vi "GetConfiguredSounds.vi"(11 "File":string="soundconfig.xml") -> (1 "Sound Cluster":T2={"Start"={"total number of samples/ch"=31680, "sound format"={"sample rate (S/s)"=11025.0, "number of channels"=1, "bits per sample"=16}, "data"=[{"t0"=timestamp(0 s since 1904-01-01), "dt"=9.070294784580499e-05, "Y"=array[31680 elements]}], "Volume"=100.0}, "Stop"={"total number of samples/ch"=27648, "sound format"={"sample rate (S/s)"=11025.0, "number of channels"=1, "bits per sample"=16}, "data"=[{"t0"=timestamp(0 s since 1904-01-01), "dt"=9.070294784580499e-05, "Y"=array[27648 elements]}], "Volume"=100.0}, "Uh-Oh"={"total number of samples/ch"=29952, "sound format"={"sample rate (S/s)"=11025.0, "number of channels"=1, "bits per sample"=16}, "data"=[{"t0"=timestamp(0 s since 1904-01-01), "dt"=9.070294784580499e-05, "Y"=array[29952 elements]}], "Volume"=88.46153846153847}, "PreMatch"={"total number of samples/ch"=225792, "sound format"={"sample rate (S/s)"=44100.0, "number of channels"=2, "bits per sample"=16}, "data"=[{"t0"=timestamp(0 s since 1904-01-01), "dt"=2.2675736961451248e-05, "Y"=array[225792 elements]}, {"t0"=timestamp(0 s since 1904-01-01), "dt"=2.2675736961451248e-05, "Y"=array[225792 elements]}], "Volume"=75.38461538461539}, "Hurry-Up"={"total number of samples/ch"=0, "sound format"={"sample rate (S/s)"=0.0, "number of channels"=0, "bits per sample"=0}, "data"=[], "Volume"=0.0}}, 3 "Settings Cluster":T1)   [LabVIEW 2013]
uses:
  Sound Info.ctl
  <vilib>/sound2/lvsound2.llb/Sound Data Format.ctl
  <vilib>/Utility/sysdir.llb/System Directory Type.ctl
  <vilib>/Utility/xml.llb/Read From XML File(string).vi
panel:
  in  "stop":bool
  out "output cluster":T1
  in  "Tab Control":enum32{"Page 1", "Page 2"}(tab)
  in  "Test Hurry Up Sound":bool
  in  "Load Hurry Up Sound":bool
  in  "Hurry Up Sound Volume":dbl(slide)=88.46153846153847 scale=0.0..100.0
  in  "Hurry Up Sound":path=path "C:/ProgramData/FLL/sounds/TimeToRun.wav"
  in  "Test Pre-Match Sound":bool
  in  "Load Pre-Match Sound":bool
  in  "Pre-Match Coundown Sound Volume":dbl(slide)=88.46153846153847 scale=0.0..100.0
  in  "Pre-Match Countdown Sound":path=path "Z:/Code/LabVIEW/FLL 2.1/sounds/FOGHORN.wav"
  in  "Test Uh-Oh Sound":bool
  in  "Load Uh-Oh Sound":bool
  in  "Uh-Oh Sound Volume":dbl(slide)=88.46153846153847 scale=0.0..100.0
  in  "Uh-Oh Sound Path":path=path "Z:/Code/LabVIEW/FLL 2.1/sounds/FOGHORN.wav"
  in  "Test Stop Sound":bool
  in  "Load Stop Sound":bool
  in  "Stop Sound Volume":dbl(slide)=100.0 scale=0.0..100.0
  in  "Stop Sound Path":path=path "Z:/Code/LabVIEW/FLL 2.1/sounds/BUZZER.wav"
  in  "Test Start Sound":bool
  in  "Load Start Sound":bool
  in  "Start Sound Volume":dbl(slide)=100.0 scale=0.0..100.0
  in  "Start Sound Path":path=path "Z:/Code/LabVIEW/FLL 2.1/sounds/CHARGE.wav"
  in  "Master Volume":dbl(slide)=100.0 min=1.0 scale=0.0..100.0
  in  "Secondary (s)":dbl
  in  "Primary (s)":dbl=150.0
  in  "Pre-Primary (s)":dbl
  # "5"
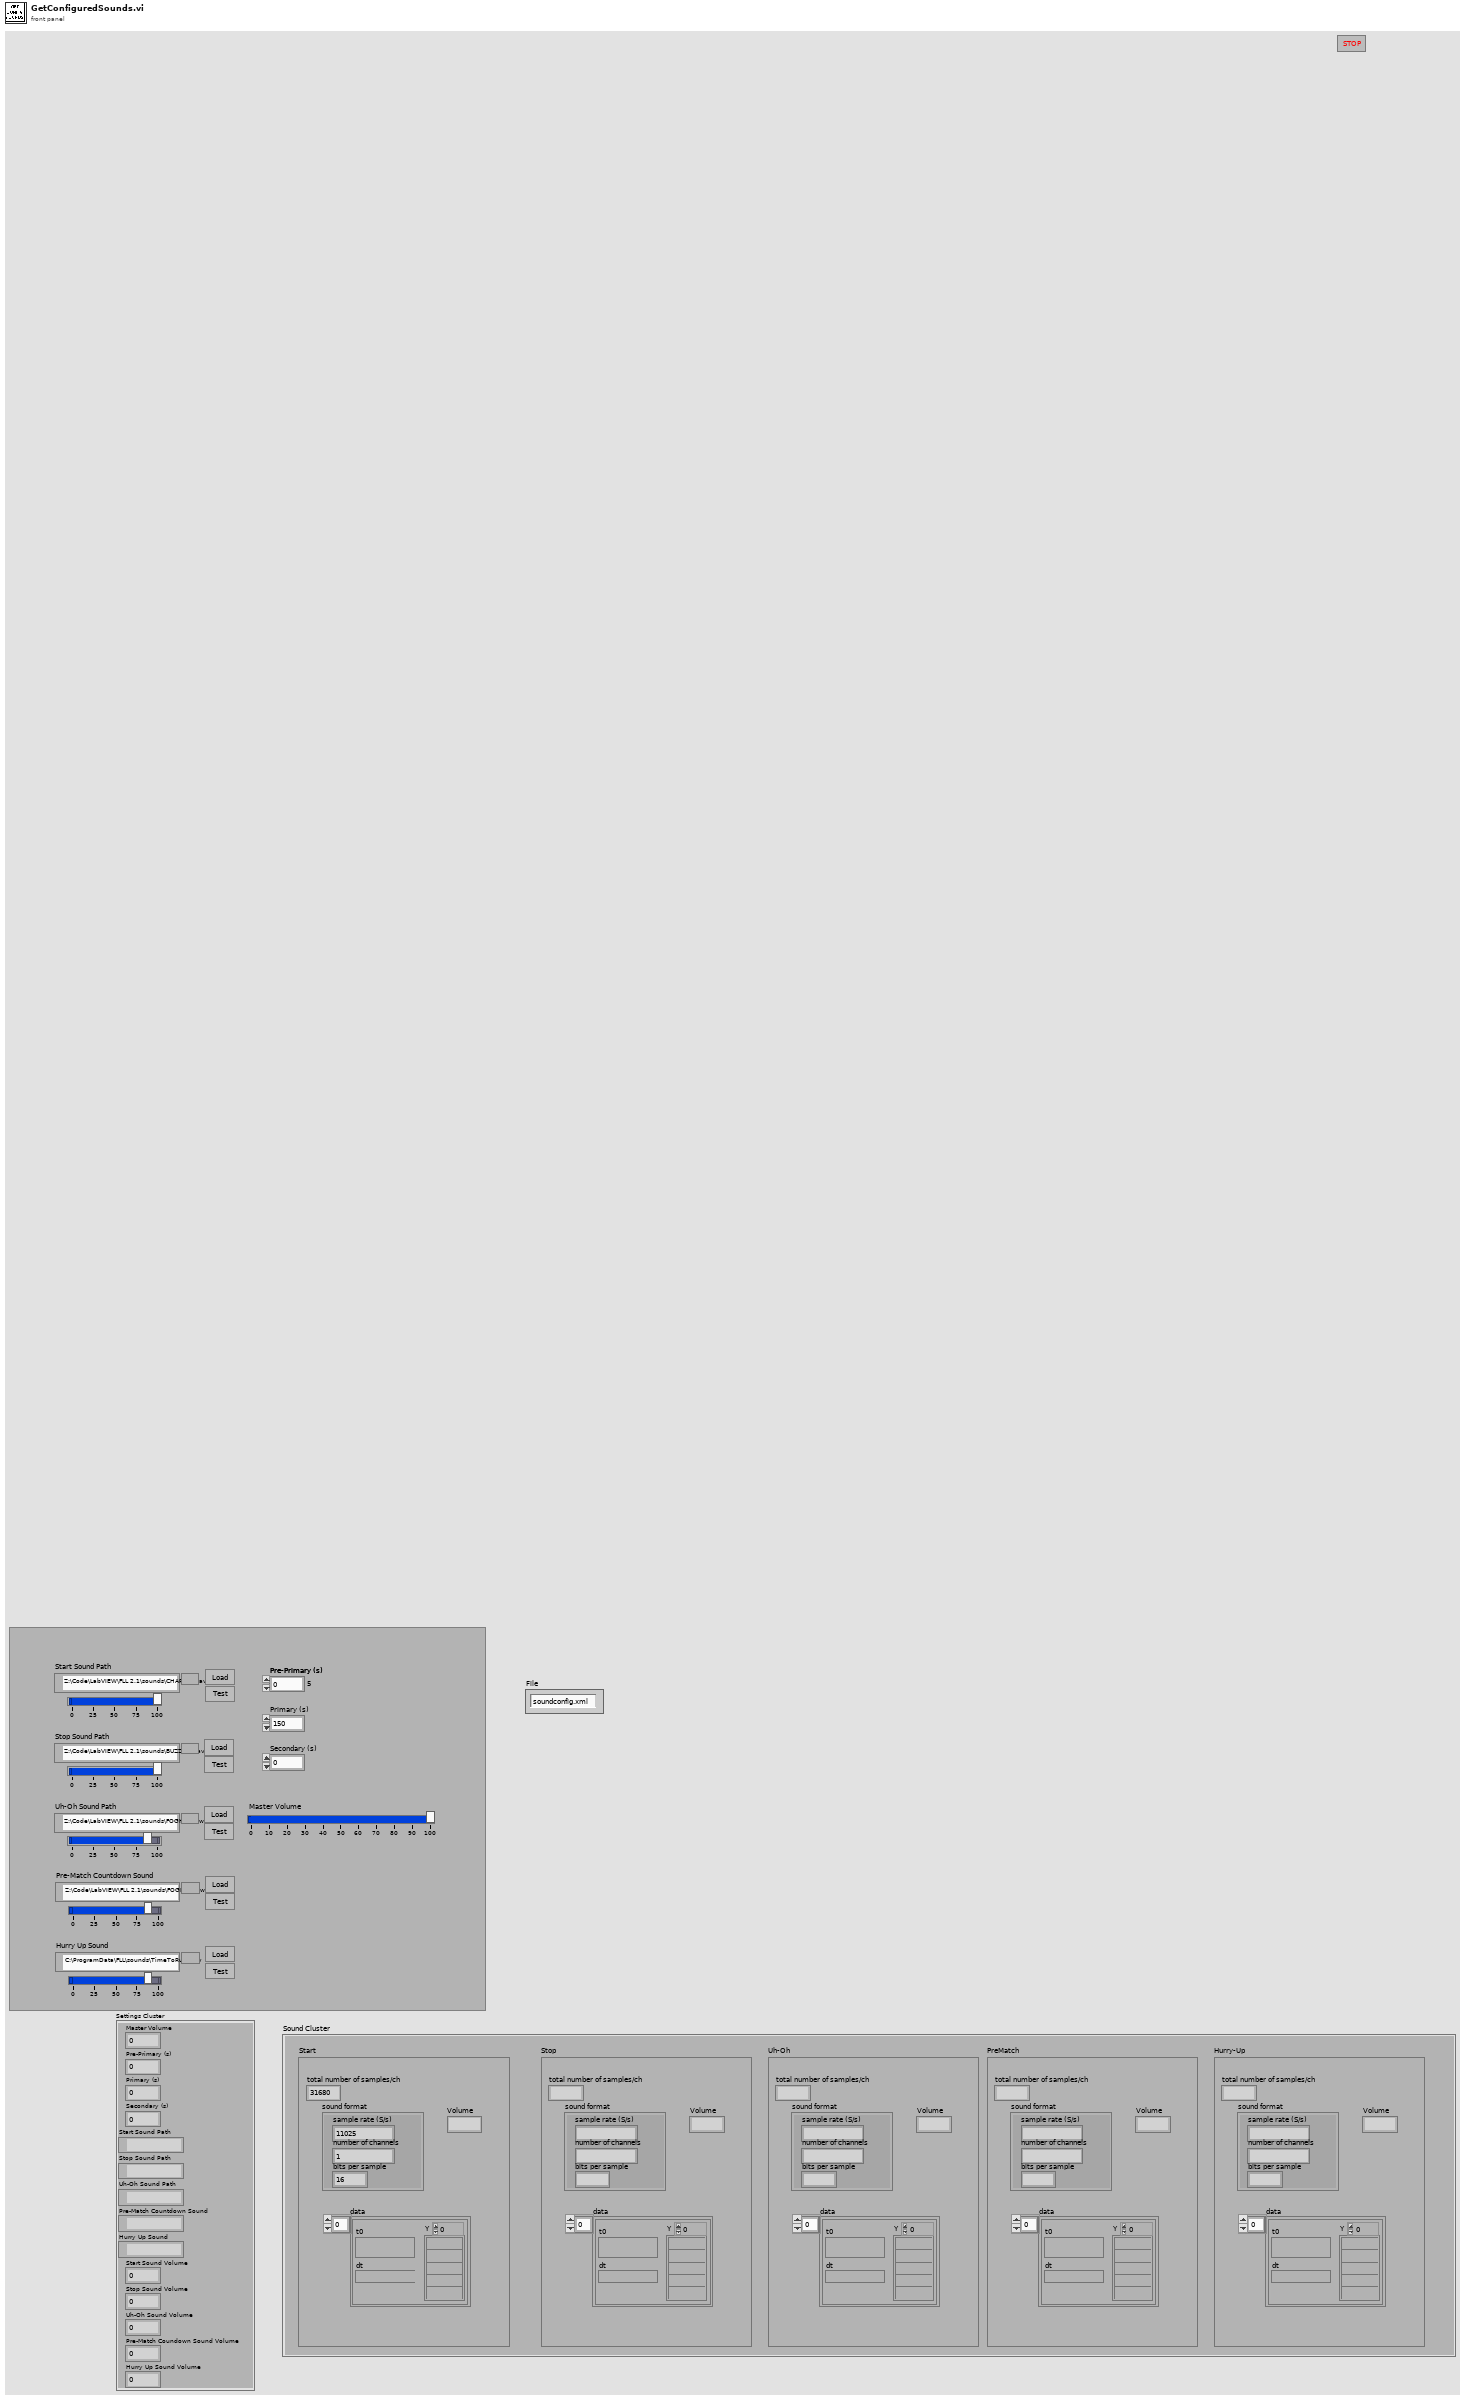
[diagram p1: front panel]
types:
  T1 = cluster{"Master Volume":dbl, "Pre-Primary (s)":dbl, "Primary (s)":dbl, "Secondary (s)":dbl, "Start Sound Path":path, "Stop Sound Path":path, "Uh-Oh Sound Path":path, "Pre-Match Countdown Sound":path, "Hurry Up Sound":path, "Start Sound Volume":dbl, "Stop Sound Volume":dbl, "Uh-Oh Sound Volume":dbl, "Pre-Match Coundown Sound Volume":dbl, "Hurry Up Sound Volume":dbl}
  T2 = typedef "Sound Info.ctl" = cluster{"Start":cluster{"total number of samples/ch":u32, "sound format":T3, "data":waveform(dbl)[], "Volume":dbl}, "Stop":cluster{"total number of samples/ch":u32, "sound format":T3, "data":waveform(dbl)[], "Volume":dbl}, "Uh-Oh":cluster{"total number of samples/ch":u32, "sound format":T3, "data":waveform(dbl)[], "Volume":dbl}, "PreMatch":cluster{"total number of samples/ch":u32, "sound format":T3, "data":waveform(dbl)[], "Volume":dbl}, "Hurry-Up":cluster{"total number of samples/ch":u32, "sound format":T3, "data":waveform(dbl)[], "Volume":dbl}}
  T3 = typedef "Sound Data Format.ctl" = cluster{"sample rate (S/s)":dbl, "number of channels":i32, "bits per sample":i32}
  T4 = typedef "System Directory Type.ctl" = i32
  T5 = cluster{"total number of samples/ch":u32, "sound format":T3, "data":waveform(dbl)[], "Volume":dbl}
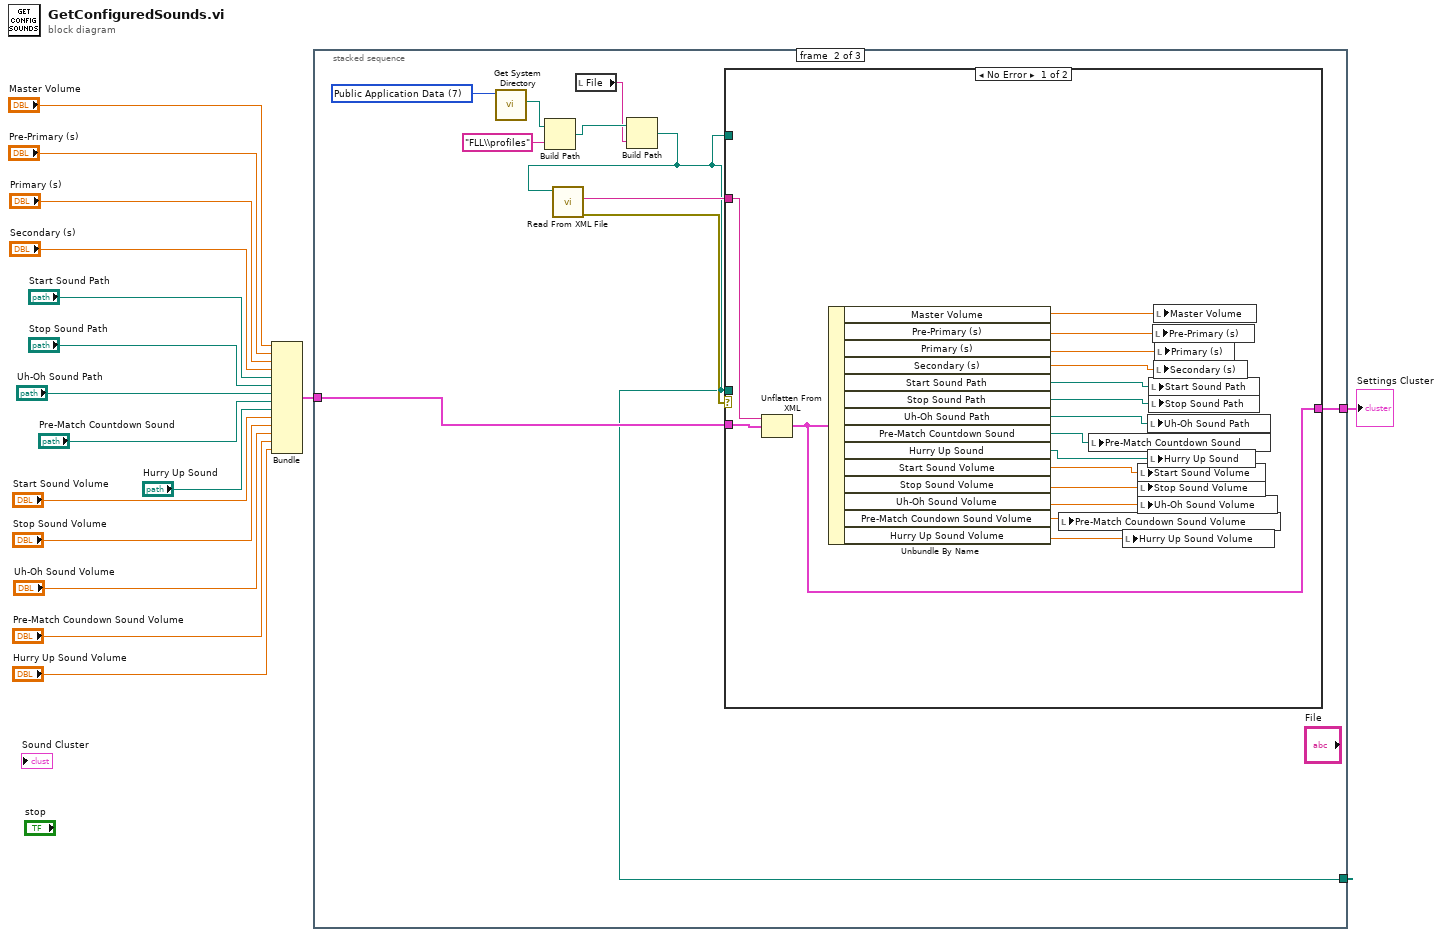
[diagram p0: block diagram]
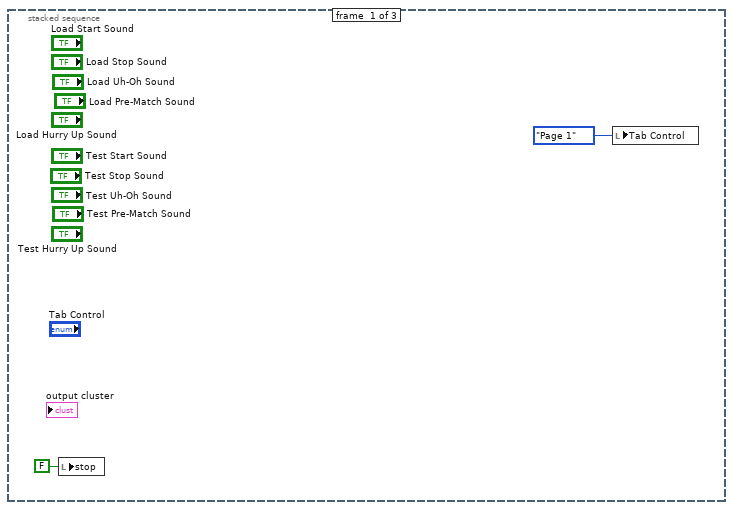
[diagram p2: hidden frame]
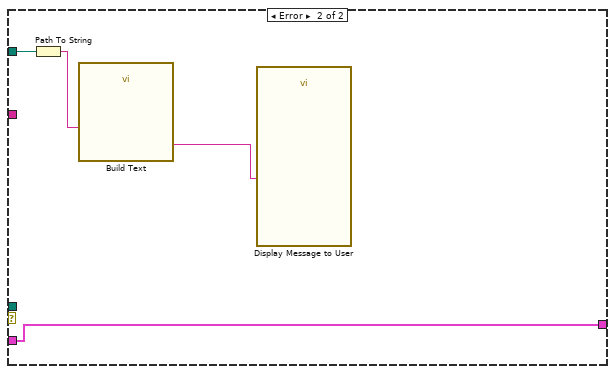
[diagram p3: hidden frame]
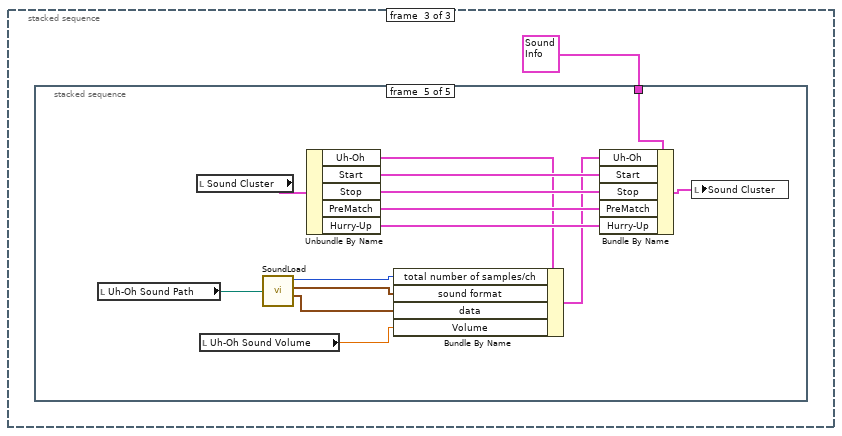
[diagram p4: hidden frame]
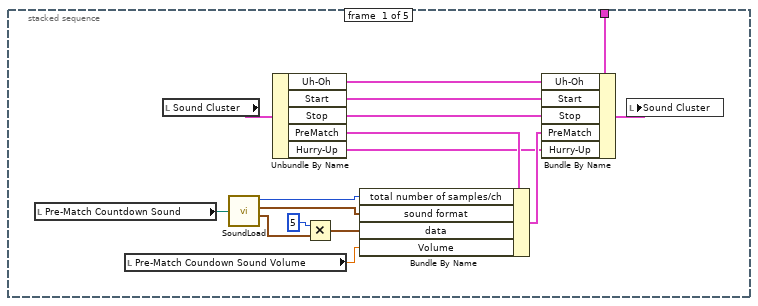
[diagram p5: hidden frame]
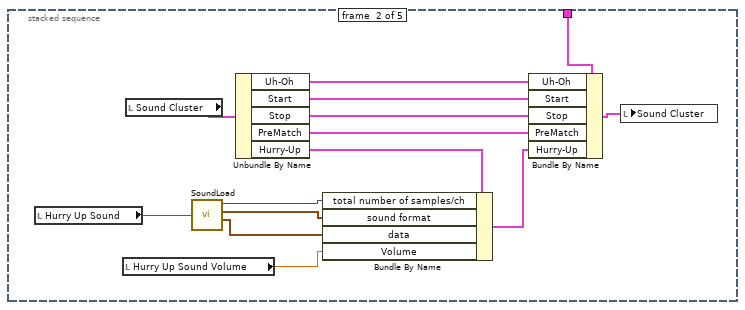
[diagram p6: hidden frame]
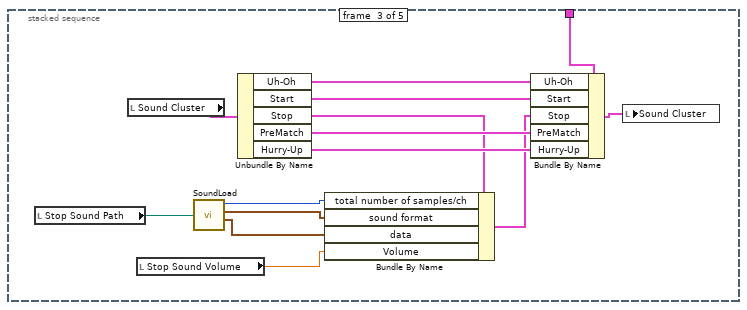
[diagram p7: hidden frame]
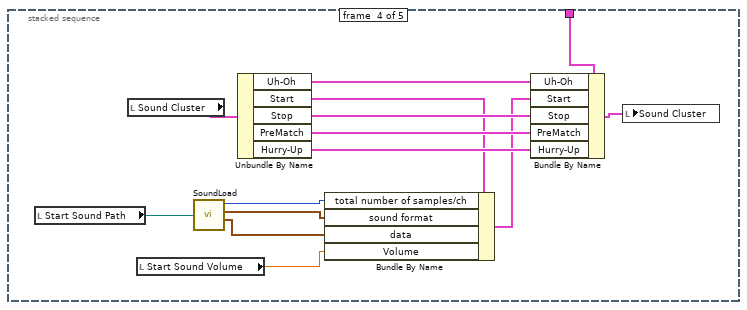
[diagram p8: hidden frame]
diagram:
  n1 = Bundle("Master Volume"="Master Volume", "Pre-Primary (s)"="Pre-Primary (s)", "Primary (s)"="Primary (s)", "Secondary (s)"="Secondary (s)", "Start Sound Path"="Start Sound Path", "Stop Sound Path"="Stop Sound Path", "Uh-Oh Sound Path"="Uh-Oh Sound Path", "Pre-Match Countdown Sound"="Pre-Match Countdown Sound", "Hurry Up Sound"="Hurry Up Sound", "Start Sound Volume"="Start Sound Volume", "Stop Sound Volume"="Stop Sound Volume", "Uh-Oh Sound Volume"="Uh-Oh Sound Volume", "Pre-Match Coundown Sound Volume"="Pre-Match Coundown Sound Volume", "Hurry Up Sound Volume"="Hurry Up Sound Volume") -> (w2:T1)  [unwired: 1 in]
  n2 = stacked-sequence {
    tunnel: w2 -> [_ w24 _]
    tunnel: [_ w19 _] -> _
    tunnel: [_ w22 _] -> w1
    frame #0 {
      n3 = local write "stop"(FALSE ("stop")) -> ()
      n4 = local write "Tab Control"(enum32{"Page 1", "Page 2"}."Page 1" ("Tab Control")) -> ()
    }
    frame #1 {
      w28 = T4 7 items=["User Home"=0, "User Desktop"=1, "User Documents"=2, "User Application Data"=3, "User Preferences"=4, "User Temporary"=5, "Public Documents"=6, "Public Application Data"=7, "Public Preferences"=8, "Public Cache"=13, "System Core Libraries"=9, "System Installed Libraries"=10, "Application Files"=11, "Boot Volume Root"=12] ("system directory type")
      n5 = call <vilib>:"Get System Directory.vi"("system directory type"=w28) -> ("system directory"=w27:path)  [unwired: 10 in]
      n6 = Build Path(base path=w27, name or relative path="FLL\\profiles") -> (appended path=w21:path)
      n7 = local read "File"() -> (w20:string)
      n8 = Build Path(base path=w21, name or relative path=w20) -> (appended path=w19:path)
      n9 = call-poly <vilib>:"Read From XML File.vi"("XML File Path"=w19) -> ("error out"=w25:errorcluster, "XML Elements"=w23:string)  [unwired: 8 in, 1 out]
      n10 = case shown="No Error" w25 {
        tunnel: w19 -> [_ _]
        tunnel: w24 -> [w45 w46]
        tunnel: w23 -> [w44 _]
        tunnel: w19 -> [_ w49]
        tunnel: [w29 w46] -> w22
        frame No Error {
          n11 = Unflatten From XML(xml string=w44, type=w45) -> (value=w29:T1)  [unwired: 1 in, 1 out]
          n12 = Unbundle By Name(w29) -> ("Master Volume"=w43:dbl, "Pre-Primary (s)"=w42:dbl, "Primary (s)"=w41:dbl, "Secondary (s)"=w40:dbl, "Start Sound Path"=w39:path, "Stop Sound Path"=w38:path, "Uh-Oh Sound Path"=w37:path, "Pre-Match Countdown Sound"=w36:path, "Hurry Up Sound"=w35:path, "Start Sound Volume"=w34:dbl, "Stop Sound Volume"=w33:dbl, "Uh-Oh Sound Volume"=w32:dbl, "Pre-Match Coundown Sound Volume"=w31:dbl, "Hurry Up Sound Volume"=w30:dbl)
          n13 = local write "Pre-Match Coundown Sound Volume"(w31) -> ()
          n14 = local write "Pre-Match Countdown Sound"(w36) -> ()
          n15 = local write "Hurry Up Sound Volume"(w30) -> ()
          n16 = local write "Start Sound Volume"(w34) -> ()
          n17 = local write "Stop Sound Volume"(w33) -> ()
          n18 = local write "Uh-Oh Sound Volume"(w32) -> ()
          n19 = local write "Uh-Oh Sound Path"(w37) -> ()
          n20 = local write "Hurry Up Sound"(w35) -> ()
          n21 = local write "Start Sound Path"(w39) -> ()
          n22 = local write "Stop Sound Path"(w38) -> ()
          n23 = local write "Pre-Primary (s)"(w42) -> ()
          n24 = local write "Master Volume"(w43) -> ()
          n25 = local write "Secondary (s)"(w40) -> ()
          n26 = local write "Primary (s)"(w41) -> ()
        }
        frame Error {
          n27 = Path To String(path=w49) -> (string=w48:string)
          n28 = call "Build Text"("configfile"=w48) -> ("Result"=w47:string)  [unwired: 13 in, 1 out]
          n29 = call "Display Message to User"("Message"=w47) -> ()  [unwired: 9 in, 2 out]
        }
      }
    }
    frame #2 {
      n30 = stacked-sequence {
        tunnel: T2 {"Start"={"total number of samples/ch"=0, "sound format"={"sample rate (S/s)"=0.0, "number of channels"=0, "bits per sample"=0}, "data"=[], "Volume"=0.0}, "Stop"={"total number of samples/ch"=0, "sound format"={"sample rate (S/s)"=0.0, "number of channels"=0, "bits per sample"=0}, "data"=[], "Volume"=0.0}, "Uh-Oh"={"total number of samples/ch"=0, "sound format"={"sample rate (S/s)"=0.0, "number of channels"=0, "bits per sample"=0}, "data"=[], "Volume"=0.0}, "PreMatch"={"total number of samples/ch"=0, "sound format"={"sample rate (S/s)"=0.0, "number of channels"=0, "bits per sample"=0}, "data"=[], "Volume"=0.0}, "Hurry-Up"={"total number of samples/ch"=0, "sound format"={"sample rate (S/s)"=0.0, "number of channels"=0, "bits per sample"=0}, "data"=[], "Volume"=0.0}} ("Sound Info") -> [w65 w79 w93 w107 w121]
        frame #0 {
          n31 = local read "Pre-Match Countdown Sound"() -> (w56:path)
          n32 = local read "Pre-Match Coundown Sound Volume"() -> (w55:dbl)
          n33 = local read "Sound Cluster"() -> (w66:T2)
          n34 = call "SoundLoad.vi"("Sound File"=w56) -> ("total number of samples/ch"=w59:u32, "sound format"=w60:T3, "data"=w53:waveform(dbl)[])  [unwired: 1 out]
          n35 = Unbundle By Name(w66) -> ("Uh-Oh"=w57:T5, "Start"=w64:T5, "Stop"=w63:T5, "PreMatch"=w62:T5, "Hurry-Up"=w51:T5)
          n36 = Multiply(x=5, y=w53) -> (x*y=w52:waveform(dbl)[])
          n37 = Bundle By Name(cluster=w62, "total number of samples/ch"=w59, "sound format"=w60, "data"=w52, "Volume"=w55) -> (w61:T5)
          n38 = Bundle By Name(cluster=w65, "Uh-Oh"=w57, "Start"=w64, "Stop"=w63, "PreMatch"=w61, "Hurry-Up"=w51) -> (w58:T2)
          n39 = local write "Sound Cluster"(w58) -> ()
        }
        frame #1 {
          n40 = local read "Hurry Up Sound"() -> (w72:path)
          n41 = local read "Hurry Up Sound Volume"() -> (w71:dbl)
          n42 = local read "Sound Cluster"() -> (w80:T2)
          n43 = call "SoundLoad.vi"("Sound File"=w72) -> ("total number of samples/ch"=w75:u32, "sound format"=w76:T3, "data"=w67:waveform(dbl)[])  [unwired: 1 out]
          n44 = Unbundle By Name(w80) -> ("Uh-Oh"=w73:T5, "Start"=w78:T5, "Stop"=w77:T5, "PreMatch"=w70:T5, "Hurry-Up"=w69:T5)
          n45 = Bundle By Name(cluster=w69, "total number of samples/ch"=w75, "sound format"=w76, "data"=w67, "Volume"=w71) -> (w68:T5)
          n46 = Bundle By Name(cluster=w79, "Uh-Oh"=w73, "Start"=w78, "Stop"=w77, "PreMatch"=w70, "Hurry-Up"=w68) -> (w74:T2)
          n47 = local write "Sound Cluster"(w74) -> ()
        }
        frame #2 {
          n48 = local read "Stop Sound Path"() -> (w87:path)
          n49 = local read "Sound Cluster"() -> (w94:T2)
          n50 = local read "Stop Sound Volume"() -> (w86:dbl)
          n51 = call "SoundLoad.vi"("Sound File"=w87) -> ("total number of samples/ch"=w90:u32, "sound format"=w91:T3, "data"=w81:waveform(dbl)[])  [unwired: 1 out]
          n52 = Unbundle By Name(w94) -> ("Uh-Oh"=w88:T5, "Start"=w92:T5, "Stop"=w83:T5, "PreMatch"=w85:T5, "Hurry-Up"=w84:T5)
          n53 = Bundle By Name(cluster=w83, "total number of samples/ch"=w90, "sound format"=w91, "data"=w81, "Volume"=w86) -> (w82:T5)
          n54 = Bundle By Name(cluster=w93, "Uh-Oh"=w88, "Start"=w92, "Stop"=w82, "PreMatch"=w85, "Hurry-Up"=w84) -> (w89:T2)
          n55 = local write "Sound Cluster"(w89) -> ()
        }
        frame #3 {
          n56 = local read "Start Sound Path"() -> (w102:path)
          n57 = local read "Sound Cluster"() -> (w108:T2)
          n58 = local read "Start Sound Volume"() -> (w101:dbl)
          n59 = call "SoundLoad.vi"("Sound File"=w102) -> ("total number of samples/ch"=w105:u32, "sound format"=w106:T3, "data"=w95:waveform(dbl)[])  [unwired: 1 out]
          n60 = Unbundle By Name(w108) -> ("Uh-Oh"=w103:T5, "Start"=w97:T5, "Stop"=w98:T5, "PreMatch"=w100:T5, "Hurry-Up"=w99:T5)
          n61 = Bundle By Name(cluster=w97, "total number of samples/ch"=w105, "sound format"=w106, "data"=w95, "Volume"=w101) -> (w96:T5)
          n62 = Bundle By Name(cluster=w107, "Uh-Oh"=w103, "Start"=w96, "Stop"=w98, "PreMatch"=w100, "Hurry-Up"=w99) -> (w104:T2)
          n63 = local write "Sound Cluster"(w104) -> ()
        }
        frame #4 {
          n64 = local read "Uh-Oh Sound Path"() -> (w118:path)
          n65 = local read "Sound Cluster"() -> (w122:T2)
          n66 = local read "Uh-Oh Sound Volume"() -> (w117:dbl)
          n67 = call "SoundLoad.vi"("Sound File"=w118) -> ("total number of samples/ch"=w119:u32, "sound format"=w120:T3, "data"=w113:waveform(dbl)[])  [unwired: 1 out]
          n68 = Unbundle By Name(w122) -> ("Uh-Oh"=w111:T5, "Start"=w112:T5, "Stop"=w114:T5, "PreMatch"=w116:T5, "Hurry-Up"=w115:T5)
          n69 = Bundle By Name(cluster=w111, "total number of samples/ch"=w119, "sound format"=w120, "data"=w113, "Volume"=w117) -> (w110:T5)
          n70 = Bundle By Name(cluster=w121, "Uh-Oh"=w110, "Start"=w112, "Stop"=w114, "PreMatch"=w116, "Hurry-Up"=w115) -> (w109:T2)
          n71 = local write "Sound Cluster"(w109) -> ()
        }
      }
    }
  }
  "Settings Cluster" <- w1
